vi "Altitude Composite.vi"(5 "Feet OFF/ Meters ON":bool, 7 "West ON/Std OFF":bool=TRUE, 8 "Mode":enum8{"Off", "Stby", "Hold", "Run"}(ring), 9 "Pressure mBar":dbl=840.0, 10 "O2ppm-2":u32=209400, 11 "O2ppm-1":u32=209400) -> (0 "PO2":dbl=18003.97265625, 1 "Alt Eff correct":dbl=1449.1019287109375, 2 "O2%-2":dbl=21.433300018310547, 3 "O2%-1":dbl=21.433300018310547, 4 "System Status Out":bool, 6 "Mean O2%":dbl)   [LabVIEW 2013]
doc: "Calculate altitude based on oxygen content and barometric pressure. The inputs define whether the value is calculated using the standard equation or the West equation."
uses:
  <vilib>/Analysis/NI_AALBase.lvlib
panel:
  out "P (Pa)":dbl=84000.0
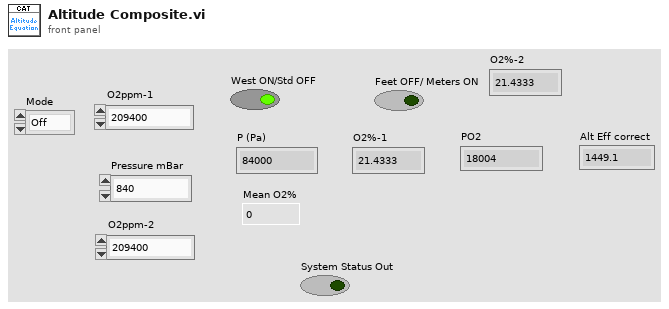
[diagram p1: front panel]
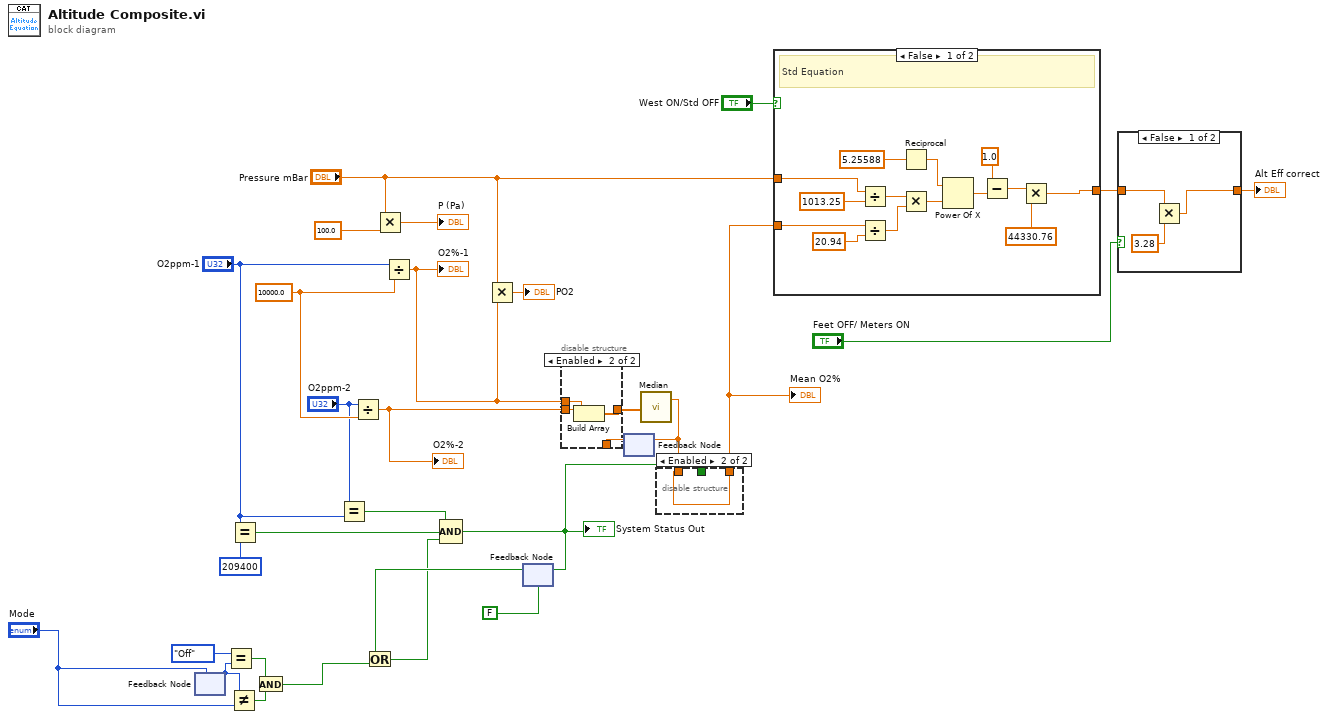
[diagram p0: block diagram]
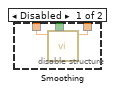
[diagram p2: hidden frame]
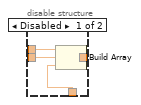
[diagram p3: hidden frame]
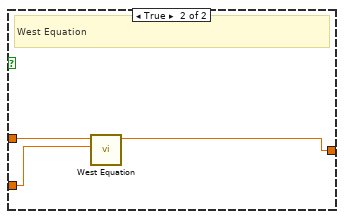
[diagram p5: hidden frame]
diagram:
  w22 = 10000.0 ("y")
  n1 = feedback #1() -> (w7:enum8{"Off", "Stby", "Hold", "Run"})  [unwired: 1 in]
  n2 = feedback-in #1("Mode") -> ()
  n3 = Equal?(x=enum8{"Off", "Stby", "Hold", "Run"}."Off", y=w7) -> (x = y?=w8:bool)
  n4 = Not Equal?(x=w7, y="Mode") -> (x != y?=w6:bool)
  n5 = Equal?(x="O2ppm-1", y=u32 209400 ("value")) -> (x = y?=w19:bool)
  n6 = And(x=w8, y=w6) -> (x .and. y?=w4:bool)
  n7 = Equal?(x="O2ppm-2", y="O2ppm-1") -> (x = y?=w18:bool)
  n8 = Divide(x="O2ppm-2", y=w22) -> (x/y=w12:dbl)
  "O2%-2" <- w12
  n9 = Multiply(x="Pressure mBar", y=100.0) -> (x*y=→"P (Pa)":dbl)
  n10 = Divide(x="O2ppm-1", y=w22) -> (x/y=w13:dbl)
  "O2%-1" <- w13
  n11 = Multiply(x="Pressure mBar", y=w13) -> (x*y=→"PO2":dbl)
  n12 = feedback #2(FALSE) -> (w3:bool)
  n13 = Or(x=w3, y=w4) -> (x .or. y?=w2:bool)
  n14 = Compound Arithmetic op=AND(w18, w19, w2) -> (w10:bool)
  "System Status Out" <- w10
  n15 = feedback-in #2(w10) -> ()
  n16 = feedback #3() -> (w15:dbl)  [unwired: 1 in]
  n17 = disable-structure shown="Enabled" {
    disable-tunnel: w15 -> [w34 _]
    disable-tunnel: [w33 w35] -> w14
    disable-tunnel: w13 -> [w32 w37]
    disable-tunnel: w12 -> [w31 w36]
    frame Disabled {
      n18 = Build Array(w32, w31, w34) -> (w33:dbl[])
    }
    frame Enabled {
      n19 = Build Array(w37, w36) -> (w35:dbl[])
    }
  }
  n20 = call <vilib>:"Median.vi"("X"=w14) -> ("median"=w11:dbl)  [unwired: 1 out]
  n21 = feedback-in #3(w11) -> ()
  n22 = disable-structure shown="Enabled" {
    disable-tunnel: w11 -> [w40 w41]
    disable-tunnel: w10 -> [w39 _]
    disable-tunnel: [w38 w41] -> w9
    frame Disabled {
      n23 = call "Smoothing.vi"("Warming up?"=w39, "O2%"=w40) -> ("Mean O2%"=w38:dbl)  [unwired: 9 in]
    }
    frame Enabled {
    }
  }
  "Mean O2%" <- w9
  n24 = case shown="False" "West ON/Std OFF" {
    tunnel: "Pressure mBar" -> [w44 w58]
    tunnel: w9 -> [w43 w57]
    tunnel: [w42 w56] -> w30
    frame False {
      # "Std Equation"
      n25 = Divide(x=w44, y=1013.25) -> (x/y=w48:dbl)
      n26 = Divide(x=w43, y=20.94) -> (x/y=w47:dbl)
      n27 = Reciprocal(x=5.25588 ("y")) -> (1/x=w55:dbl)
      n28 = Multiply(x=w48, y=w47) -> (x*y=w51:dbl)
      n29 = Power Of X(1:w51, 2:w55) -> (0:w50:dbl)
      n30 = Subtract(x=1.0, y=w50) -> (x-y=w54:dbl)
      n31 = Multiply(x=w54, y=44330.76) -> (x*y=w42:dbl)
    }
    frame True {
      # "West Equation"
      n32 = call "West Equation.vi"("O2%"=w57, "P (mb)"=w58) -> ("Altitude (m)"=w56:dbl)  [unwired: 9 in]
    }
  }
  n33 = case shown="False" "Feet OFF/ Meters ON" {
    tunnel: w30 -> [w61 w62]
    tunnel: [w59 w62] -> w24
    frame False {
      n34 = Multiply(x=w61, y=3.28) -> (x*y=w59:dbl)
    }
    frame True {
    }
  }
  "Alt Eff correct" <- w24
